vi "Car Wash.vi"(7 "Start":bool, 9 "stop":bool, 10 "Car Position Slider":u8(slide) max=3 scale=0.0..4.0, 11 "Wash Options":T1) -> (0 "error out":errorcluster, 1 "Elapsed Time":dbl format="%0.2f", 2 "Car Wash Indicators":T2, 3 "Wash Entry":bool)   [LabVIEW 2018]
uses:
  Controls/Car Wash Indicators.ctl
  Controls/Wash Options.ctl
  Controls/Car Wash States.ctl
panel:
  out "Array of Control Labels":string[](array[string])
  # "Entry Console"
  # "Car Wash Display"
  # "Car Position Simulation"
  # "Pre-Soak\nH-P Wash\nL-P Wax\nSpot Free Rinse"
  # "Underbody Wash\nBug Remover"
  # "Tire Shine\nAir Dry"
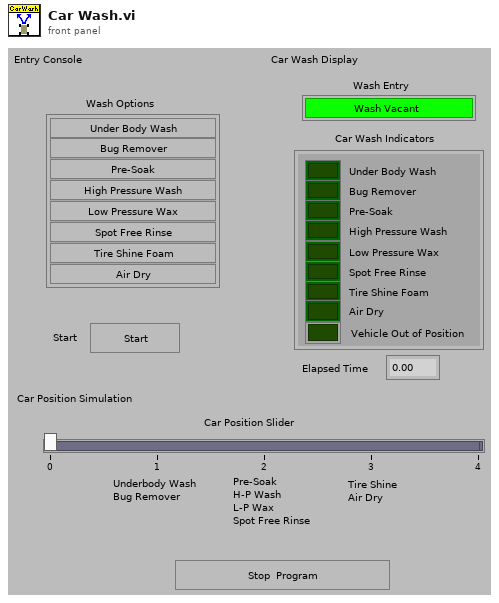
[diagram p1: front panel]
types:
  T1 = typedef "Wash Options.ctl" = cluster{"Underbody Wash":bool, "Bug Remover":bool, "Pre-Soak":bool, "High Pressure Wash":bool, "Low Pressure Wax":bool, "Spot Free Rinse":bool, "Tire Shine Foam":bool, "Air Dry":bool}
  T2 = typedef "Car Wash Indicators.ctl" = cluster{"Under Body Wash":bool, "Bug Remover":bool, "Pre-Soak":bool, "High Pressure Wash":bool, "Low Pressure Wax":bool, "Spot Free Rinse":bool, "Tire Shine Foam":bool, "Air Dry":bool, "Vehicle Out of Position":bool}
  T3 = typedef "Car Wash States.ctl" = enum16{"Initialize", "Customer Select", "Create Wash Process", "Reset Timer", "Under Body Wash", "Bug Remover", "Pre-Soak", "High Pressure Wash", "Low Pressure Wax", "Spot Free Rinse", "Tire Shine Foam", "Air Dry", "Out of Position", "Wash Finished", "Stop"}
  T4 = enum8{"Enabled", "Disabled", "Disabled and Grayed Out"}
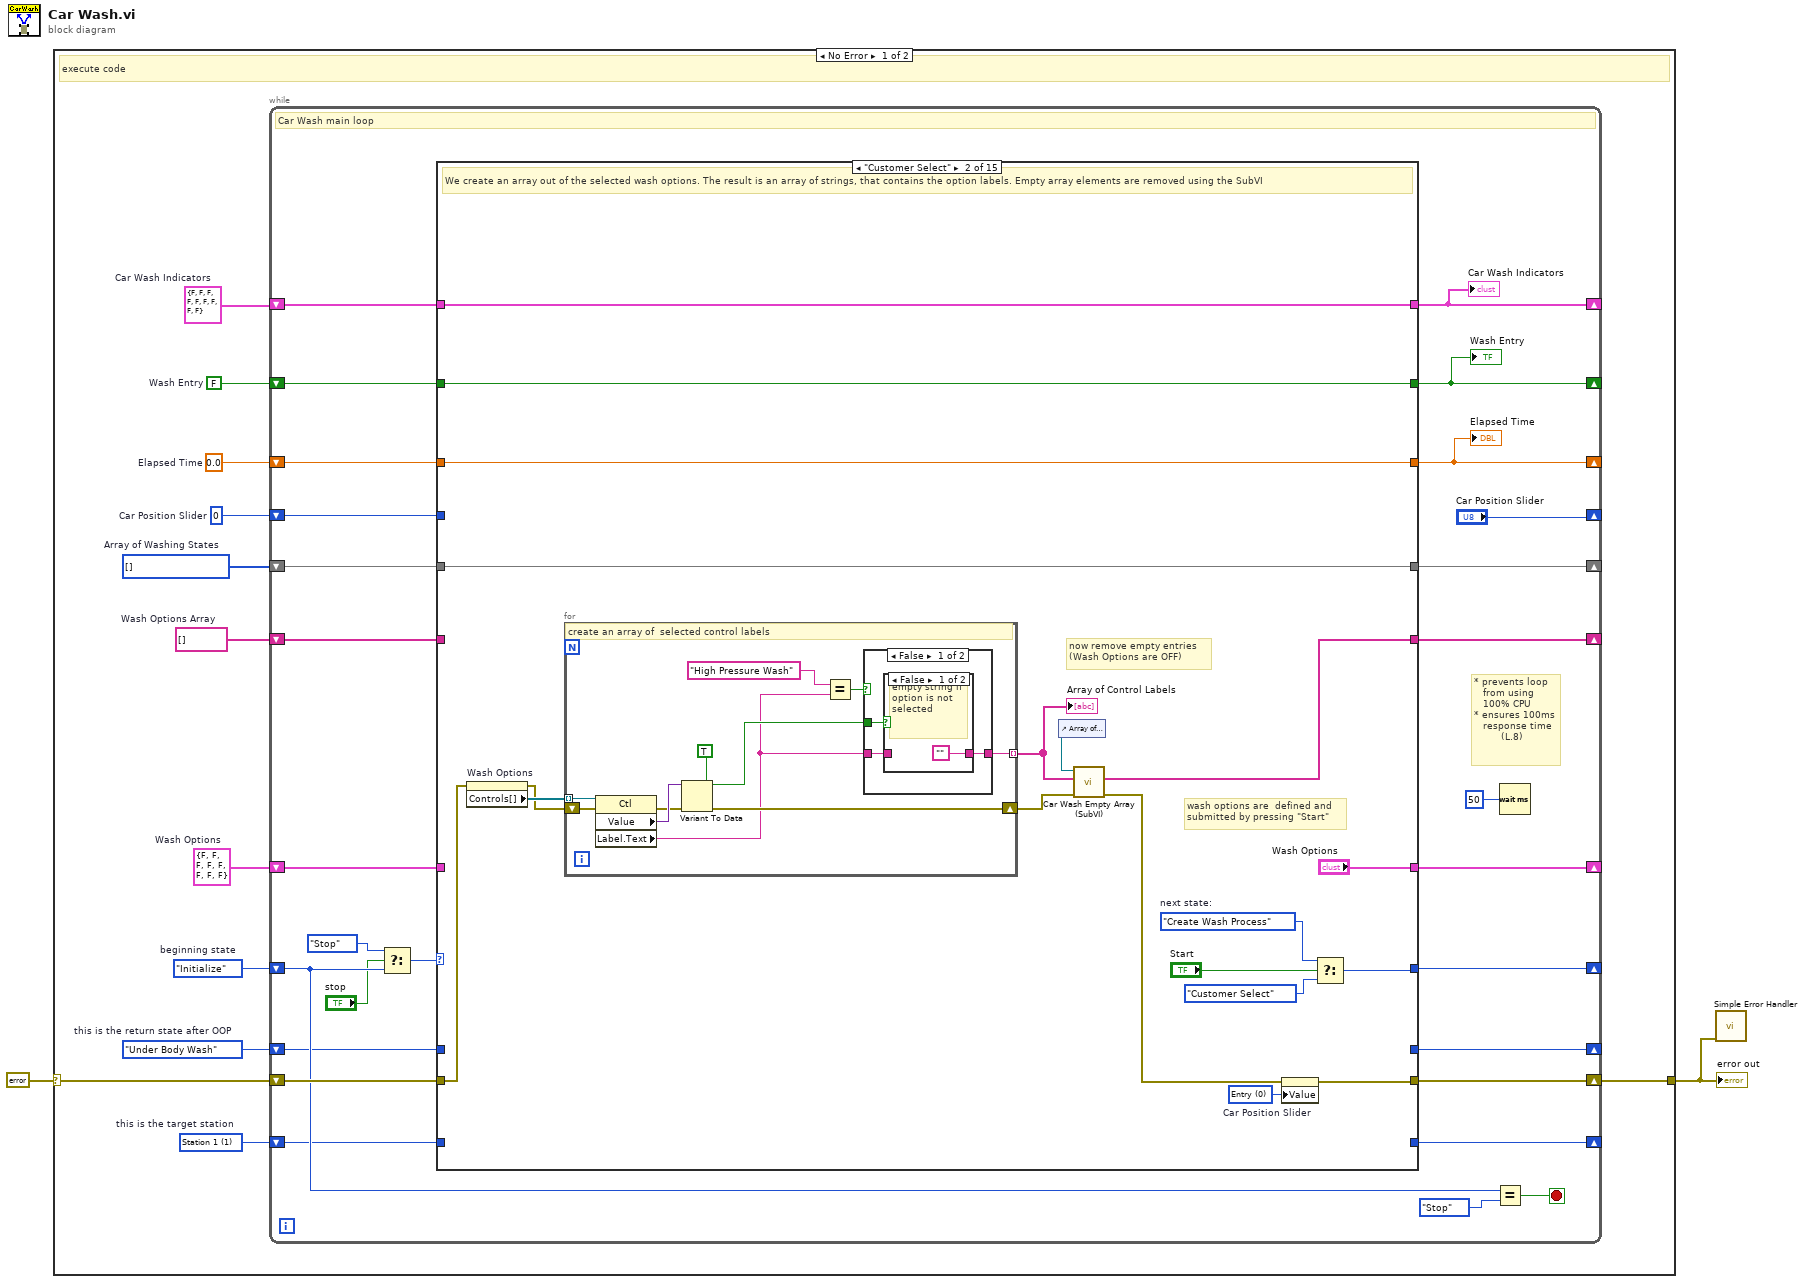
[diagram p0: block diagram]
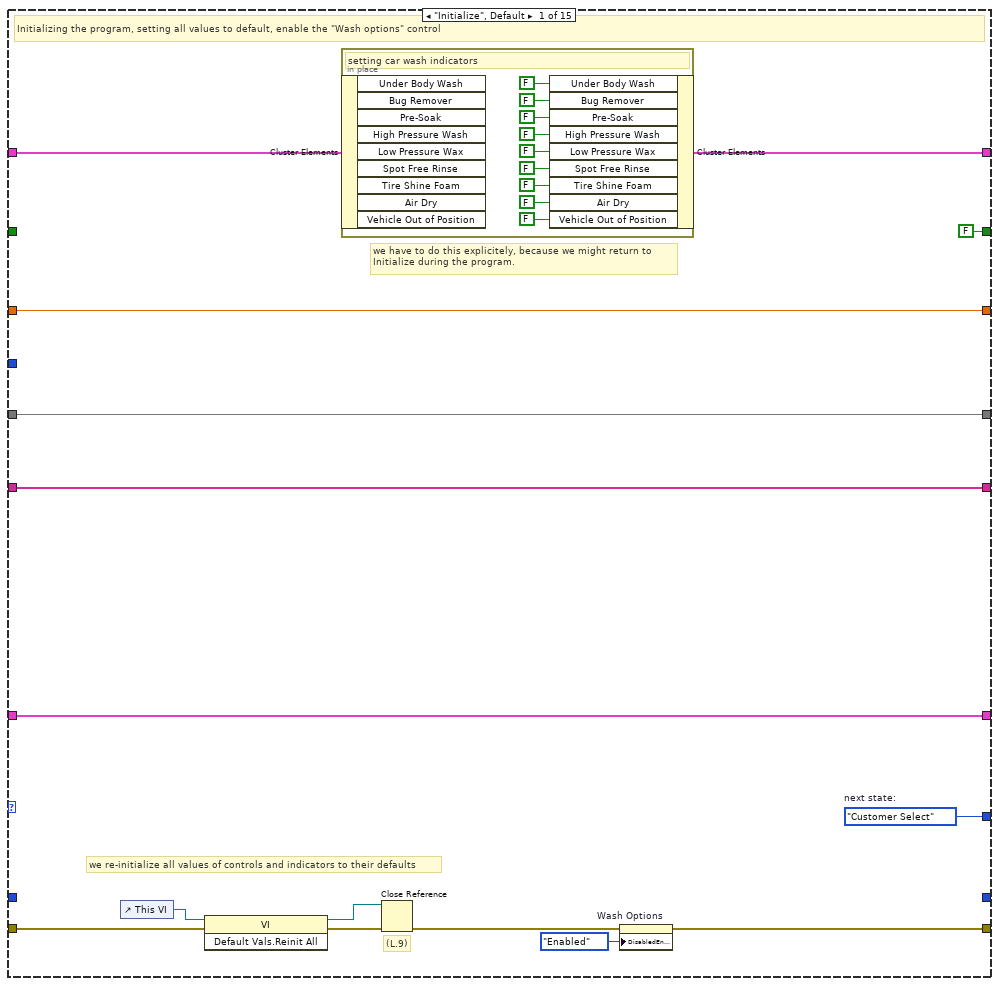
[diagram p2: hidden frame]
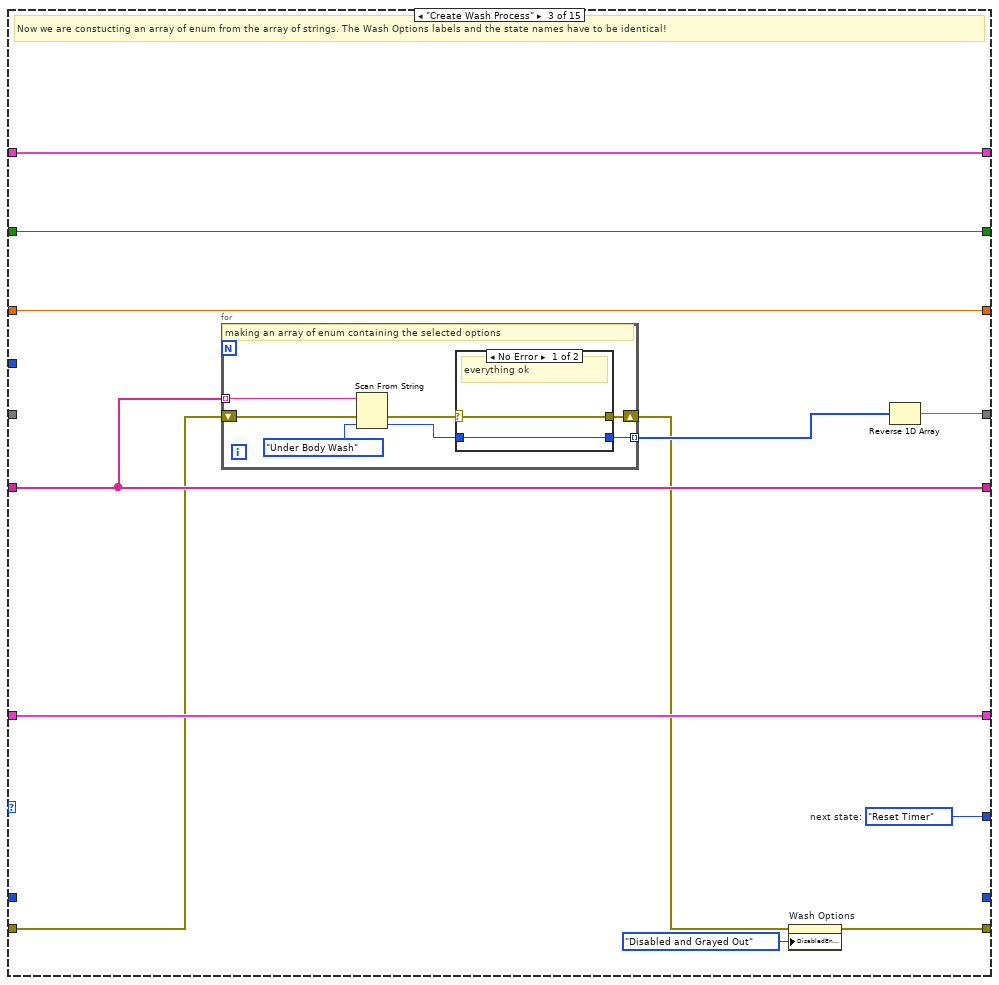
[diagram p5: hidden frame]
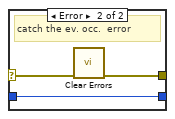
[diagram p6: hidden frame]
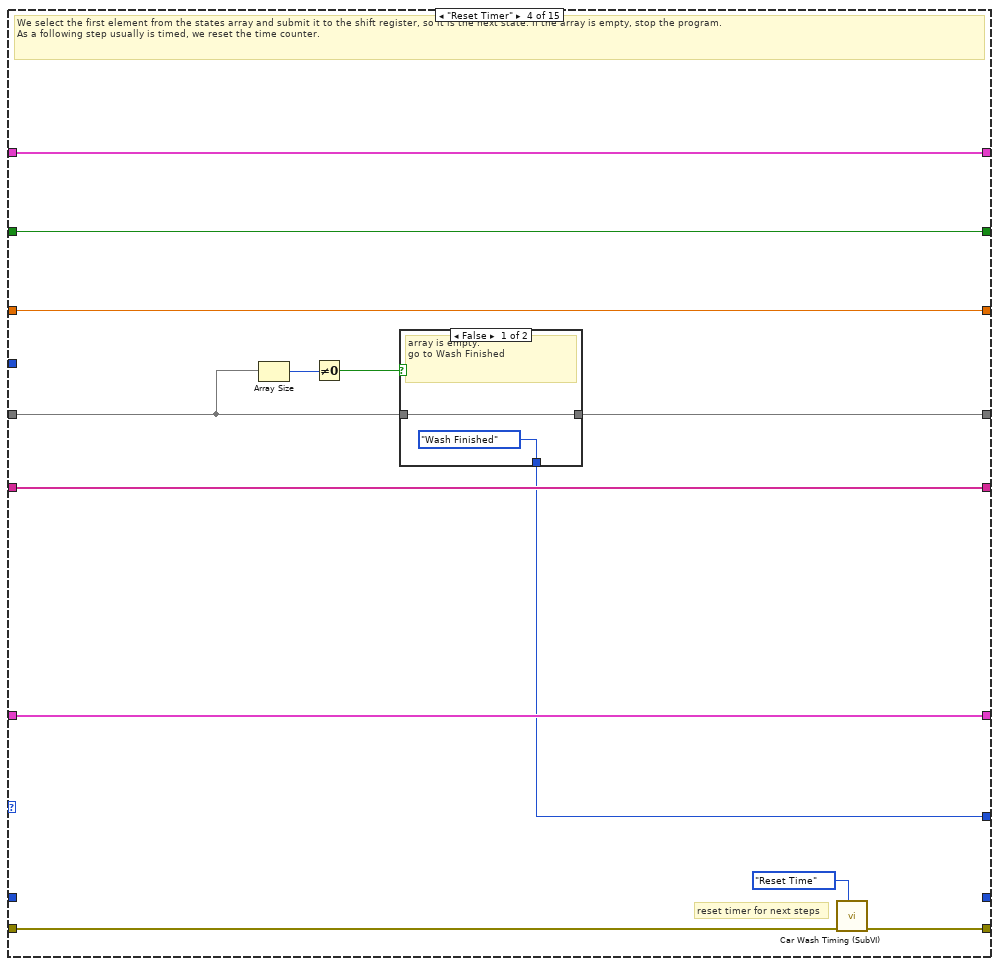
[diagram p7: hidden frame]
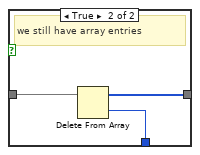
[diagram p8: hidden frame]
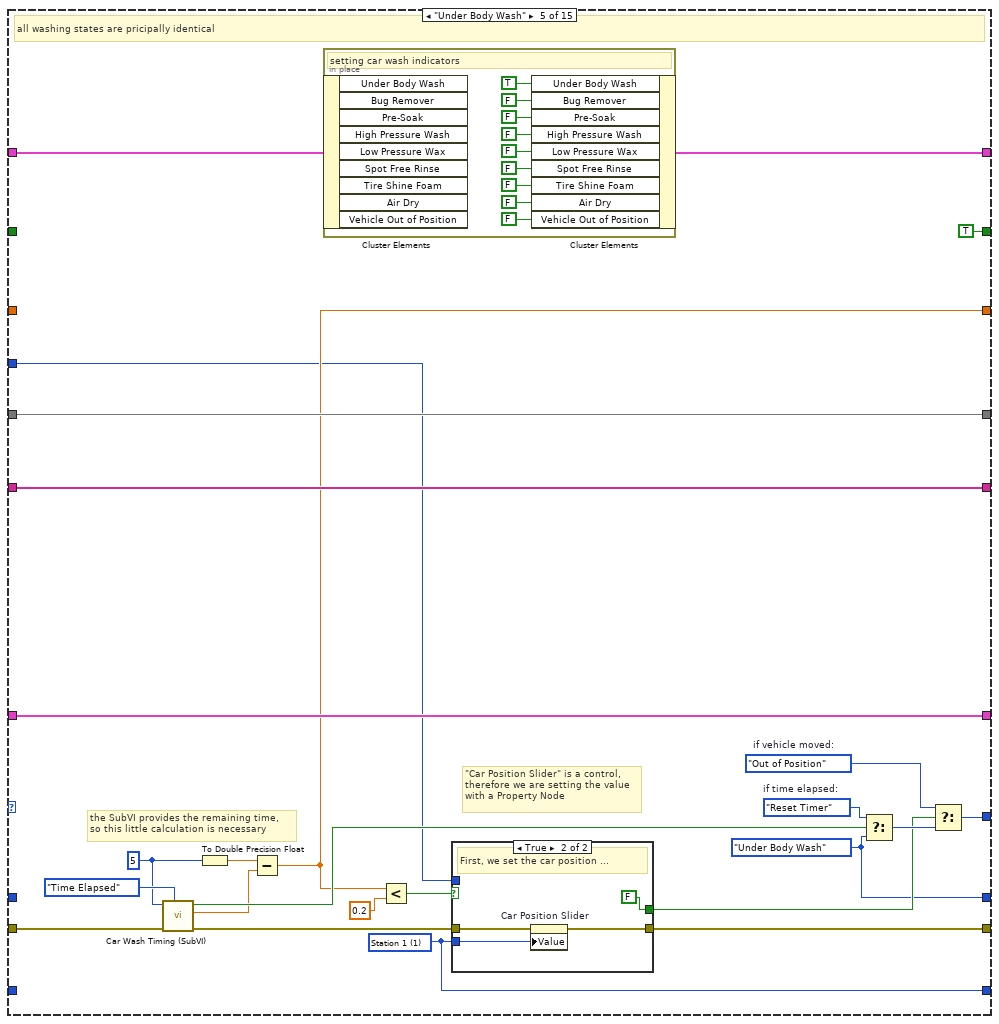
[diagram p9: hidden frame]
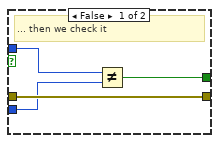
[diagram p10: hidden frame]
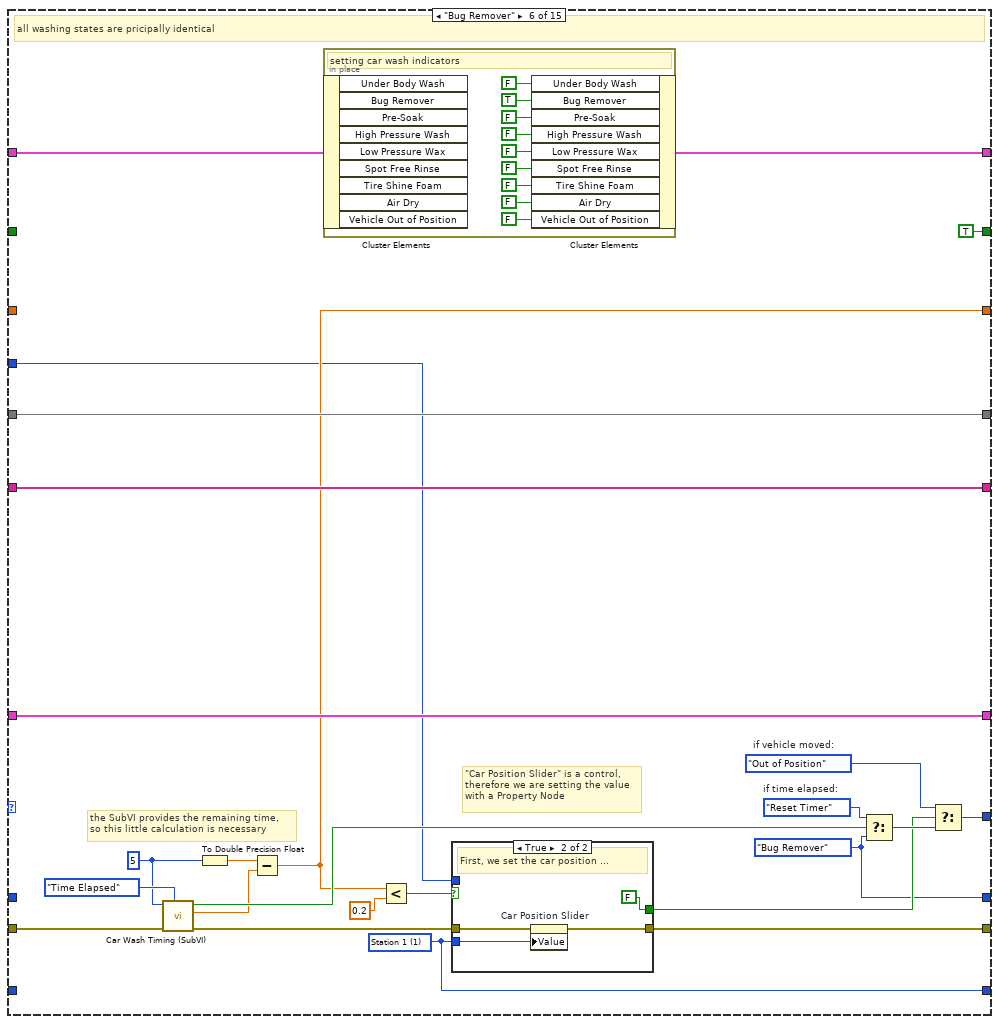
[diagram p11: hidden frame]
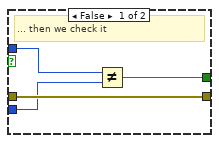
[diagram p12: hidden frame]
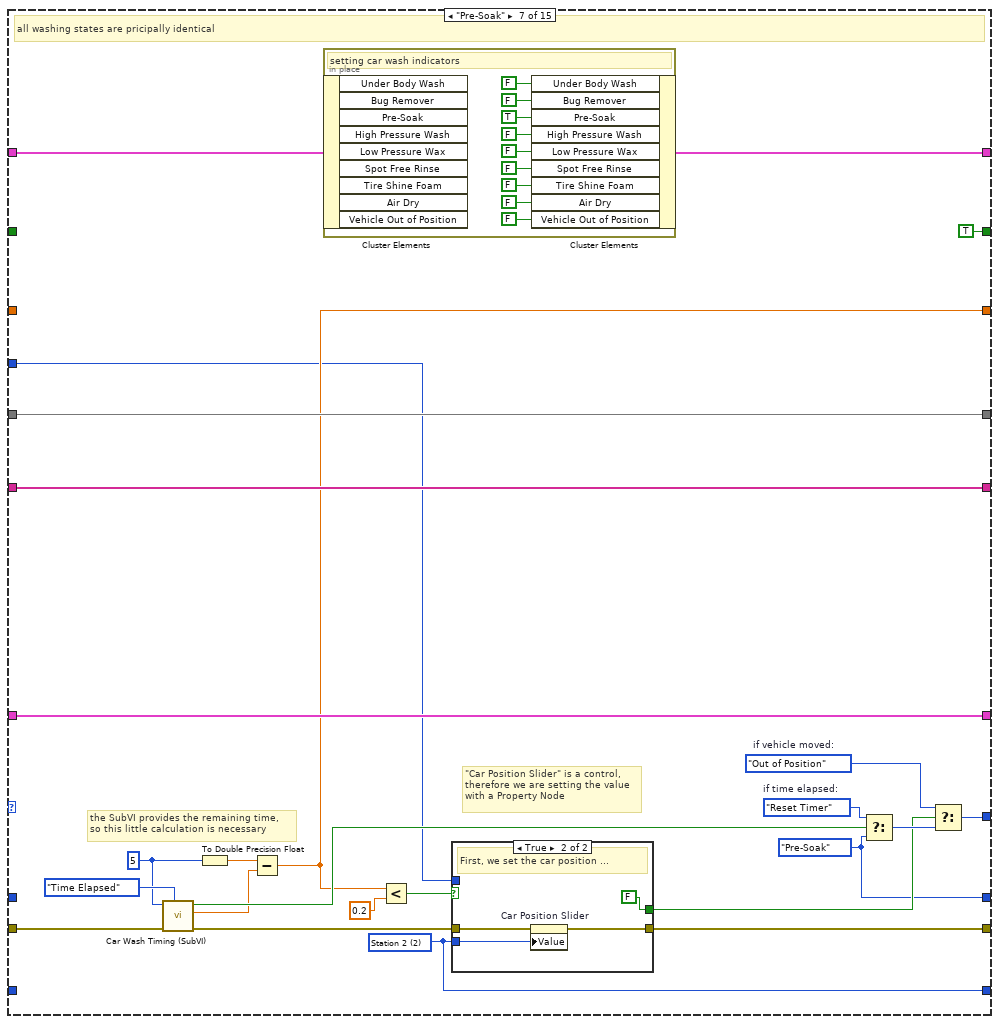
[diagram p13: hidden frame]
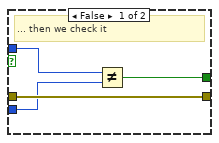
[diagram p14: hidden frame]
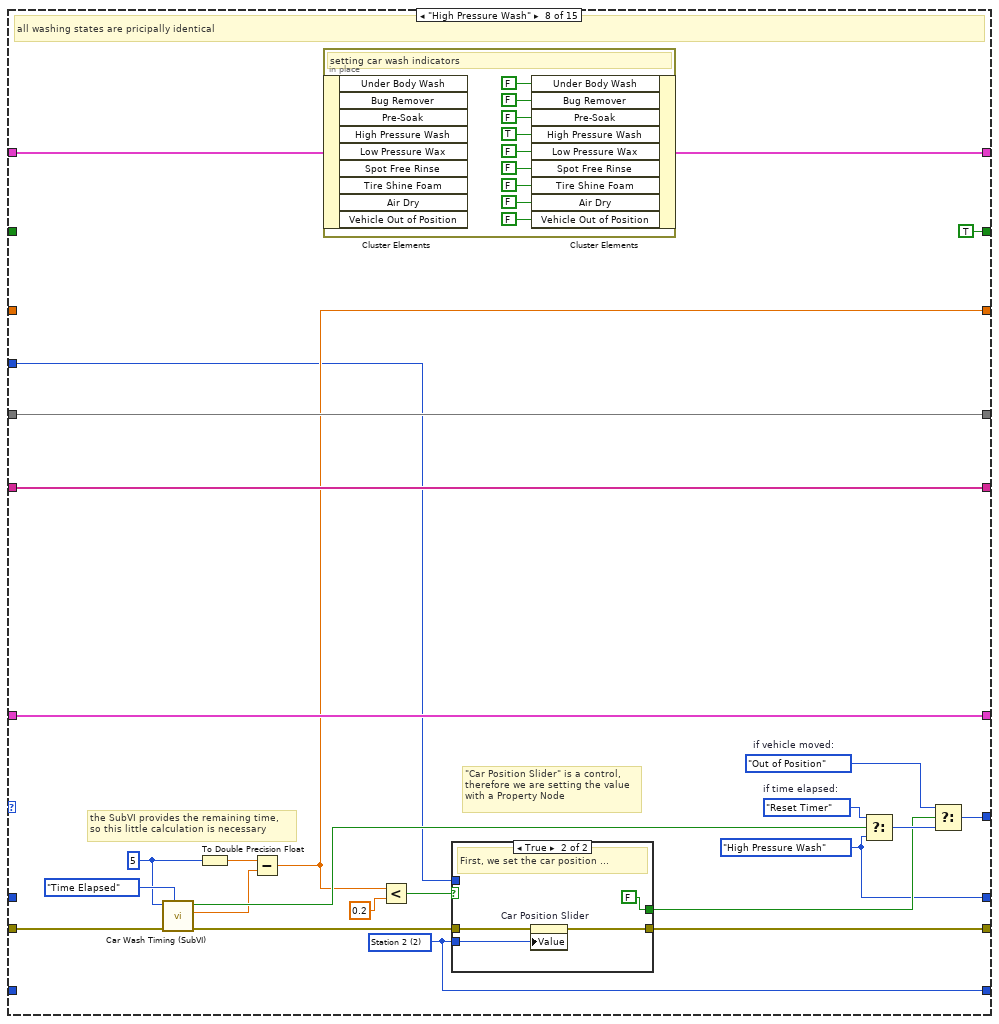
[diagram p15: hidden frame]
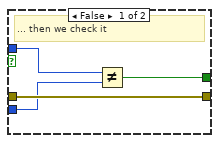
[diagram p16: hidden frame]
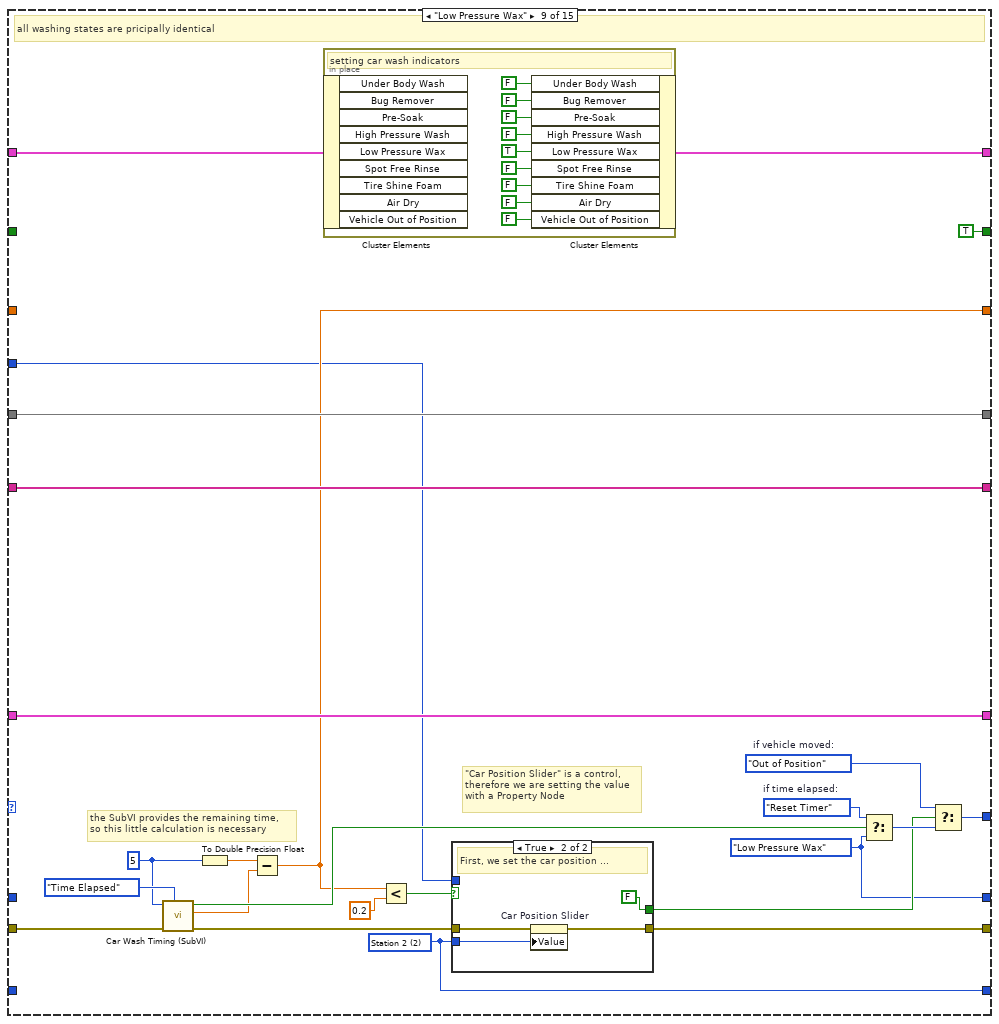
[diagram p17: hidden frame]
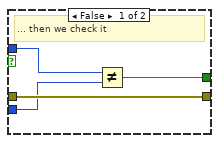
[diagram p18: hidden frame]
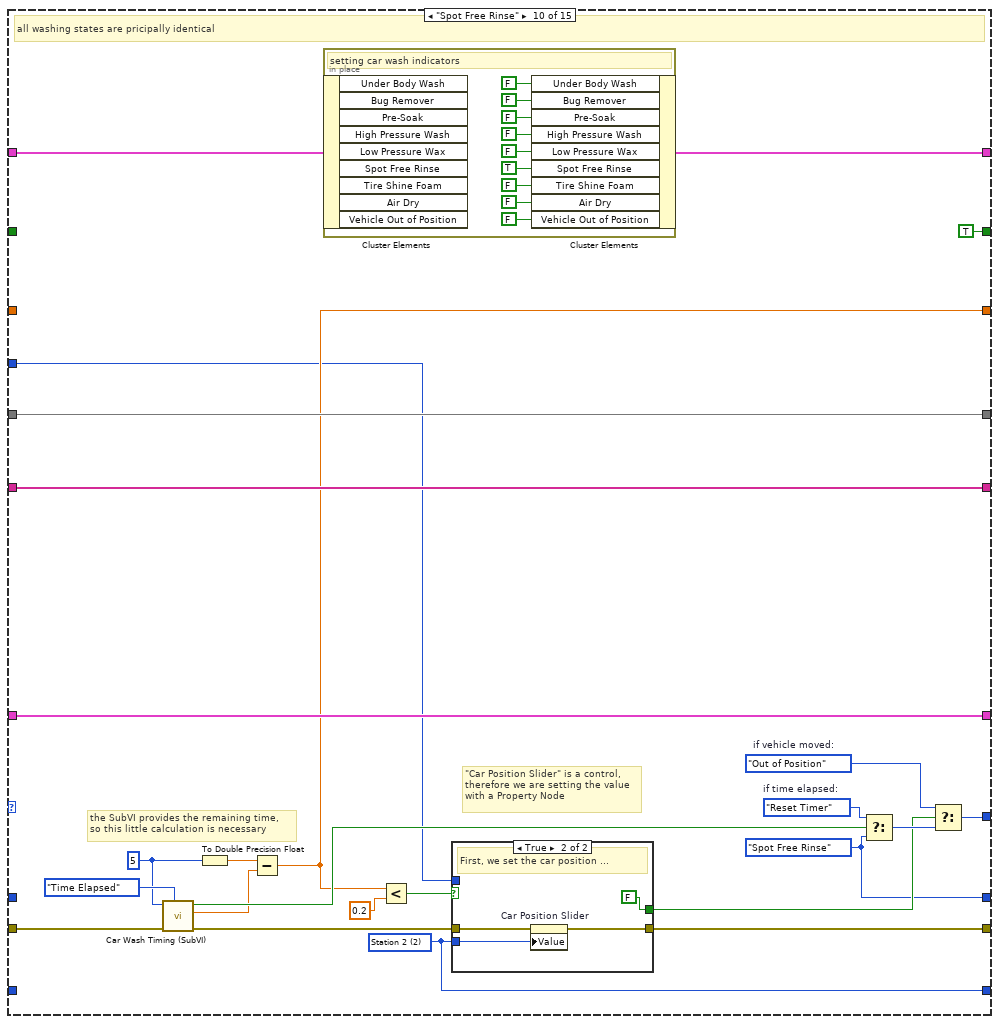
[diagram p19: hidden frame]
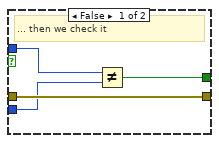
[diagram p20: hidden frame]
diagram:
  n1 = case shown="No Error" errorcluster {"status"=FALSE, "code"=0, "source"=""} ("error in (no error)") {
    selector: errorcluster {"status"=FALSE, "code"=0, "source"=""} ("error in (no error)") -> [w14 w544]
    tunnel: [w13 w544] -> w1
    frame No Error {
      w3 = u8 1 items=["Entry", "Station 1", "Station 2", "Station 3", "Exit"]  # this is the target station
      w4 = Car_Wash_States."Under Body Wash"  # this is the return state after OOP
      w6 = T3[] [] items=["Initialize", "Customer Select", "Create Wash Process", "Reset Timer", "Under Body Wash", "Bug Remover", "Pre-Soak", "High Pressure Wash", "Low Pressure Wax", "Spot Free Rinse", "Tire Shine Foam", "Air Dry", "Out of Position", "Wash Finished", "Stop"]  # Array of Washing States
      w7 = string[] []  # Wash Options Array
      w8 = 0.0  # Elapsed Time
      w9 = FALSE  # Wash Entry
      w10 = T2 {"Under Body Wash"=FALSE, "Bug Remover"=FALSE, "Pre-Soak"=FALSE, "High Pressure Wash"=FALSE, "Low Pressure Wax"=FALSE, "Spot Free Rinse"=FALSE, "Tire Shine Foam"=FALSE, "Air Dry"=FALSE, "Vehicle Out of Position"=FALSE}  # Car Wash Indicators
      w5 = u8 0  # Car Position Slider
      w11 = T1 {"Underbody Wash"=FALSE, "Bug Remover"=FALSE, "Pre-Soak"=FALSE, "High Pressure Wash"=FALSE, "Low Pressure Wax"=FALSE, "Spot Free Rinse"=FALSE, "Tire Shine Foam"=FALSE, "Air Dry"=FALSE}  # Wash Options
      w12 = Car_Wash_States."Initialize"  # beginning state
      # "execute code"
      n2 = while {
        shift-right: [w41] -> w13
        shift-left: w14 -> [w42]
        shift-right: [w25] -> _
        shift-left: w12 -> [w31]
        shift-right: [w37] -> _
        shift-left: w11 -> [w38]
        shift-right: ["Car Position Slider"] -> _
        shift-left: w5 -> [w19]
        shift-right: [w34] -> _
        shift-left: w10 -> [w35]
        shift-right: [w32] -> _
        shift-left: w9 -> [w33]
        shift-right: [w26] -> _
        shift-left: w8 -> [w27]
        shift-right: [w23] -> _
        shift-left: w7 -> [w22]
        shift-right: [w21] -> _
        shift-left: w6 -> [w20]
        shift-right: [w18] -> _
        shift-left: w4 -> [w17]
        shift-right: [w16] -> _
        shift-left: w3 -> [w15]
        stop <- w40 stop-if-true
        # "* prevents loop\n   from using\n   100% CPU\n* ensures 100ms\n   response time\n         (L.8)"
        # "Car Wash main loop"
        n3 = Select(t=Car_Wash_States."Stop", s="stop", f=w31) -> (s? t:f=w30:T3)
        n4 = case shown="\"Customer Select\"" w30 {
          tunnel: w42 -> [w54 w75 w108 w138 w154 w196 w238 w280 w322 w364 w406 w448 w488 w511 w534]
          tunnel: [w43 w69 w104 w139 w149 w191 w233 w275 w317 w359 w401 w443 w488 w505 w529] -> w41
          tunnel: w38 -> [w53 _ w111 w136 w169 w211 w253 w295 w337 w379 w421 w463 w494 w518 w542]
          tunnel: [w53 "Wash Options" w111 w136 w169 w211 w253 w295 w337 w379 w421 w463 w494 w518 w542] -> w37
          tunnel: [w44 w85 w114 w133 w167 w209 w251 w293 w335 w377 w419 w461 w492 w516 w539] -> w34
          tunnel: w35 -> [w45 w85 w114 w133 w168 w210 w252 w294 w336 w378 w420 w462 w493 w517 _]
          tunnel: [FALSE ("Wash Entry") w84 w113 w135 TRUE ("Wash Entry") TRUE ("Wash Entry") TRUE ("Wash Entry") TRUE ("Wash Entry") TRUE ("Wash Entry") TRUE ("Wash Entry") TRUE ("Wash Entry") TRUE ("Wash Entry") TRUE ("Wash Entry") TRUE ("Wash Entry") FALSE ("Wash Entry")] -> w32
          tunnel: w33 -> [_ w84 w113 w135 _ _ _ _ _ _ _ _ _ _ _]
          tunnel: [w52 w83 w112 w134 w152 w194 w236 w278 w320 w362 w404 w446 w487 0.0 ("Elapsed Time") 0.0 ("Elapsed Time")] -> w26
          tunnel: w27 -> [w52 w83 w112 w134 _ _ _ _ _ _ _ _ w487 _ _]
          tunnel: [w51 w82 w110 w130 w157 w199 w241 w283 w325 w367 w409 w451 w486 w512 Car_Wash_States."Stop" ("t")] -> w25
          tunnel: w19 -> [_ _ _ _ w148 w190 w232 w274 w316 w358 w400 w442 w483 _ _]
          tunnel: [w48 w71 w109 w132 w159 w201 w243 w285 w327 w369 w411 w453 w490 w510 string[] [] ("Wash Options Array")] -> w23
          tunnel: w22 -> [w48 _ w109 w132 w159 w201 w243 w285 w327 w369 w411 w453 w490 w510 _]
          tunnel: [w47 w70 w106 w131 w158 w200 w242 w284 w326 w368 w410 w452 w489 w509 w531] -> w21
          tunnel: w20 -> [w47 w70 _ w127 w158 w200 w242 w284 w326 w368 w410 w452 w489 w509 _]
          tunnel: [_ _ _ _ w146 w188 w230 w272 w314 w356 w398 w440 w484 _ _] -> w18
          tunnel: w17 -> [_ _ _ _ _ _ _ _ _ _ _ _ w484 _ _]
          tunnel: [_ _ _ _ w145 w187 w229 w271 w313 w355 w397 w439 w481 _ _] -> w16
          tunnel: w15 -> [_ _ _ _ _ _ _ _ _ _ _ _ w481 _ _]
          frame "Initialize", Default {
            w51 = Car_Wash_States."Customer Select"  # next state:
            # "we have to do this explicitely, because we might return to\nInitialize during the program."
            # "we re-initialize all values of controls and indicators to their defaults"
            # "(L.9)"
            # "Initializing the program, setting all values to default, enable the \"Wash options\" control"
            n5 = control-ref of="This VI"() -> (w57:refnum<vi>)
            n6 = invoke class="VI" method="Default Vals.Reinit All"(reference=w57, error in=w54) -> (reference out=w56:refnum<vi>, error out=w55:errorcluster)  [unwired: 1 in, 1 out]
            n7 = in-place {
              # "setting car wash indicators"
              n8 = in-place-cluster #1(w45) -> ()  [unwired: 9 out]
              n9 = in-place-cluster #1("Under Body Wash"=FALSE, "Bug Remover"=FALSE, "Pre-Soak"=FALSE, "High Pressure Wash"=FALSE, "Low Pressure Wax"=FALSE, "Spot Free Rinse"=FALSE, "Tire Shine Foam"=FALSE, "Air Dry"=FALSE, "Vehicle Out of Position"=FALSE) -> (w44:T2)
            }
            n10 = Close Reference(reference=w56, error in (no error)=w55) -> (error out=w50:errorcluster)
            n11 = property on="Wash Options" class="Clust (strict)"(error in=w50, "DisabledEnum"=T4."Enabled" ("Disabled")) -> (error out=w43:errorcluster)  [unwired: 1 in, 1 out]
          }
          frame "Customer Select" {
            w67 = u8 0 items=["Entry", "Station 1", "Station 2", "Station 3", "Exit"] ("Car Position Slider")
            w81 = Car_Wash_States."Create Wash Process"  # next state:
            # "wash options are  defined and\nsubmitted by pressing \"Start\""
            # "now remove empty entries\n(Wash Options are OFF)"
            # "We create an array out of the selected wash options. The result is an array of strings, that contains the option labels. Empty array elements are removed using the SubVI"
            n12 = property on="Wash Options" class="Clust (strict)"(error in=w75) -> (error out=w76:errorcluster, "Controls[]"=w77:refnum<vi>[])  [unwired: 1 in, 1 out]
            n13 = for {
              tunnel: w77 -> [w96] mode=indexing
              tunnel: [w91] -> w72 mode=indexing
              shift-right: [w89] -> w73
              shift-left: w76 -> [w90]
              # "create an array of  selected control labels"
              n14 = property on="Property Node" class="Ctl"(reference=w96, error in=w90) -> (error out=w92:errorcluster, "Value"=w95:variant, "Label.Text"=w87:string)  [unwired: 1 out]
              n15 = Variant To Data(error in=w92, type=TRUE, Variant=w95) -> (data=w93:bool, error out=w89:errorcluster)
              n16 = Equal?(x="High Pressure Wash" ("y"), y=w87) -> (x = y?=w88:bool)
              n17 = case shown="False" w88 {
                tunnel: w93 -> [w99 _]
                tunnel: [w98 w102] -> w91
                tunnel: w87 -> [w97 w102]
                frame False {
                  n18 = case shown="False" w99 {
                    tunnel: w97 -> [_ w101]
                    tunnel: ["" w101] -> w98
                    frame False {
                      # "empty string if option is not selected"
                    }
                    frame True {
                      # "put control label to array"
                    }
                  }
                }
                frame True {
                  # "This is the default\nwash and always \nadded to the \noptions"
                }
              }
            }
            "Array of Control Labels" <- w72
            n19 = control-ref of="Array of Control Labels"() -> (w74:refnum<vi>)
            n20 = call "Car Wash Empty Array (SubVI).vi"("error in (no error)"=w73, "Array in"=w72, "Array reference in"=w74) -> ("error out"=w68:errorcluster, "Array out"=w71:string[])  [unwired: 6 in, 1 out]
            n21 = property on="Car Position Slider" class="Slide (strict)"(error in=w68, "Value"=w67) -> (error out=w69:errorcluster)  [unwired: 1 in, 1 out]
            n22 = Select(t=w81, s="Start", f=Car_Wash_States."Customer Select") -> (s? t:f=w82:T3)
          }
          frame "Create Wash Process" {
            w110 = Car_Wash_States."Reset Timer"  # next state:
            # "Now we are constucting an array of enum from the array of strings. The Wash Options labels and the state names have to be identical!"
            n23 = for {
              tunnel: w109 -> [w121] mode=indexing
              tunnel: [w117] -> w107 mode=indexing
              shift-right: [w115] -> w105
              shift-left: w108 -> [w119]
              # "making an array of enum containing the selected options"
              n24 = Scan From String "Scan From String"(input string=w121, error in=w119, default 1=Car_Wash_States."Under Body Wash" ("beginning state")) -> (error out=w118:errorcluster, output 1=w116:T3)  [unwired: 2 in, 2 out]
              n25 = case shown="No Error" w118 {
                selector: w118 -> [w122 w125]
                tunnel: [w123 w126] -> w117
                tunnel: w116 -> [w123 w126]
                tunnel: [w122 w124] -> w115
                frame No Error {
                  # "everything ok"
                }
                frame Error {
                  # "catch the ev. occ.  error"
                  n26 = call <vilib>:"Clear Errors.vi"("error in (no error)"=w125) -> ("error out"=w124:errorcluster)  [unwired: 5 in, 1 out]
                }
              }
            }
            n27 = property on="Wash Options" class="Clust (strict)"(error in=w105, "DisabledEnum"=T4."Disabled and Grayed Out" ("Disabled")) -> (error out=w104:errorcluster)  [unwired: 1 in, 1 out]
            n28 = Reverse 1D Array(array=w107) -> (reversed array=w106:T3[])
          }
          frame "Reset Timer" {
            # "reset timer for next steps"
            # "We select the first element from the states array and submit it to the shift register, so it is the next state. If the array is empty, stop the program. \nAs a following step usually is timed, we reset the time counter."
            n29 = Array Size(array=w127) -> (size(s)=w129:i32)
            n30 = Not Equal To 0?(x=w129) -> (x != 0?=w128:bool)
            n31 = case shown="False" w128 {
              tunnel: [w141 w144] -> w131
              tunnel: [Car_Wash_States."Wash Finished" ("beginning state") w143] -> w130
              tunnel: w127 -> [w141 w142]
              frame False {
                # "array is empty: \ngo to Wash Finished"
              }
              frame True {
                # "we still have array entries"
                n32 = Delete From Array "Delete From Array"(array=w142) -> (deleted portion=w143:T3, array with subset deleted=w144:T3[])  [unwired: 2 in]
              }
            }
            n33 = call "Car Wash Timing (SubVI).vi"("Function"=enum16{"Reset Time", "Time Elapsed"}."Reset Time", "error in (no error)"=w138) -> ("error out"=w139:errorcluster)  [unwired: 7 in, 2 out]
          }
          frame "Under Body Wash" {
            w145 = u8 1 items=["Entry", "Station 1", "Station 2", "Station 3", "Exit"] ("Car Position Slider")
            w155 = Car_Wash_States."Out of Position"  # if vehicle moved:
            w146 = Car_Wash_States."Under Body Wash" ("t")
            w164 = Car_Wash_States."Reset Timer"  # if time elapsed:
            w160 = 5 ("Time to Wait (s)")
            # "\"Car Position Slider\" is a control,\ntherefore we are setting the value\nwith a Property Node"
            # "the SubVI provides the remaining time,\nso this little calculation is necessary"
            # "all washing states are pricipally identical"
            n34 = call "Car Wash Timing (SubVI).vi"("Function"=enum16{"Reset Time", "Time Elapsed"}."Time Elapsed", "error in (no error)"=w154, "Time to Wait (s)"=w160) -> ("error out"=w150:errorcluster, "Remaining Time"=w162:dbl, "Time elapsed ?"=w163:bool)  [unwired: 6 in]
            n35 = To Double Precision Float(number=w160) -> (double precision float=w161:dbl)
            n36 = Subtract(x=w161, y=w162) -> (x-y=w152:dbl)
            n37 = in-place {
              # "setting car wash indicators"
              n38 = in-place-cluster #2(w168) -> ()  [unwired: 9 out]
              n39 = in-place-cluster #2("Under Body Wash"=TRUE, "Bug Remover"=FALSE, "Pre-Soak"=FALSE, "High Pressure Wash"=FALSE, "Low Pressure Wax"=FALSE, "Spot Free Rinse"=FALSE, "Tire Shine Foam"=FALSE, "Air Dry"=FALSE, "Vehicle Out of Position"=FALSE) -> (w167:T2)
            }
            n40 = Less?(x=w152, y=0.2) -> (x < y?=w151:bool)
            n41 = case shown="True" w151 {
              tunnel: w150 -> [w173 w177]
              tunnel: [w173 w176] -> w149
              tunnel: w145 -> [w170 w175]
              tunnel: w148 -> [w172 _]
              tunnel: [w171 FALSE] -> w147
              frame False {
                # "... then we check it"
                n42 = Not Equal?(x=w172, y=w170) -> (x != y?=w171:bool)
              }
              frame True {
                # "First, we set the car position ..."
                n43 = property on="Car Position Slider" class="Slide (strict)"(error in=w177, "Value"=w175) -> (error out=w176:errorcluster)  [unwired: 1 in, 1 out]
              }
            }
            n44 = Select(t=w164, s=w163, f=w146) -> (s? t:f=w156:T3)
            n45 = Select(t=w155, s=w147, f=w156) -> (s? t:f=w157:T3)
          }
          frame "Bug Remover" {
            w187 = u8 1 items=["Entry", "Station 1", "Station 2", "Station 3", "Exit"] ("Car Position Slider")
            w197 = Car_Wash_States."Out of Position"  # if vehicle moved:
            w188 = Car_Wash_States."Bug Remover" ("t")
            w206 = Car_Wash_States."Reset Timer"  # if time elapsed:
            w202 = 5 ("Time to Wait (s)")
            # "\"Car Position Slider\" is a control,\ntherefore we are setting the value\nwith a Property Node"
            # "the SubVI provides the remaining time,\nso this little calculation is necessary"
            # "all washing states are pricipally identical"
            n46 = call "Car Wash Timing (SubVI).vi"("Function"=enum16{"Reset Time", "Time Elapsed"}."Time Elapsed", "error in (no error)"=w196, "Time to Wait (s)"=w202) -> ("error out"=w192:errorcluster, "Remaining Time"=w204:dbl, "Time elapsed ?"=w205:bool)  [unwired: 6 in]
            n47 = To Double Precision Float(number=w202) -> (double precision float=w203:dbl)
            n48 = Subtract(x=w203, y=w204) -> (x-y=w194:dbl)
            n49 = in-place {
              # "setting car wash indicators"
              n50 = in-place-cluster #3(w210) -> ()  [unwired: 9 out]
              n51 = in-place-cluster #3("Under Body Wash"=FALSE, "Bug Remover"=TRUE, "Pre-Soak"=FALSE, "High Pressure Wash"=FALSE, "Low Pressure Wax"=FALSE, "Spot Free Rinse"=FALSE, "Tire Shine Foam"=FALSE, "Air Dry"=FALSE, "Vehicle Out of Position"=FALSE) -> (w209:T2)
            }
            n52 = Less?(x=w194, y=0.2) -> (x < y?=w193:bool)
            n53 = case shown="True" w193 {
              tunnel: w192 -> [w215 w219]
              tunnel: [w215 w218] -> w191
              tunnel: w187 -> [w212 w217]
              tunnel: w190 -> [w214 _]
              tunnel: [w213 FALSE] -> w189
              frame False {
                # "... then we check it"
                n54 = Not Equal?(x=w214, y=w212) -> (x != y?=w213:bool)
              }
              frame True {
                # "First, we set the car position ..."
                n55 = property on="Car Position Slider" class="Slide (strict)"(error in=w219, "Value"=w217) -> (error out=w218:errorcluster)  [unwired: 1 in, 1 out]
              }
            }
            n56 = Select(t=w206, s=w205, f=w188) -> (s? t:f=w198:T3)
            n57 = Select(t=w197, s=w189, f=w198) -> (s? t:f=w199:T3)
          }
          frame "Pre-Soak" {
            w229 = u8 2 items=["Entry", "Station 1", "Station 2", "Station 3", "Exit"] ("Car Position Slider")
            w239 = Car_Wash_States."Out of Position"  # if vehicle moved:
            w230 = Car_Wash_States."Pre-Soak" ("t")
            w248 = Car_Wash_States."Reset Timer"  # if time elapsed:
            w244 = 5 ("Time to Wait (s)")
            # "\"Car Position Slider\" is a control,\ntherefore we are setting the value\nwith a Property Node"
            # "the SubVI provides the remaining time,\nso this little calculation is necessary"
            # "all washing states are pricipally identical"
            n58 = call "Car Wash Timing (SubVI).vi"("Function"=enum16{"Reset Time", "Time Elapsed"}."Time Elapsed", "error in (no error)"=w238, "Time to Wait (s)"=w244) -> ("error out"=w234:errorcluster, "Remaining Time"=w246:dbl, "Time elapsed ?"=w247:bool)  [unwired: 6 in]
            n59 = To Double Precision Float(number=w244) -> (double precision float=w245:dbl)
            n60 = Subtract(x=w245, y=w246) -> (x-y=w236:dbl)
            n61 = in-place {
              # "setting car wash indicators"
              n62 = in-place-cluster #4(w252) -> ()  [unwired: 9 out]
              n63 = in-place-cluster #4("Under Body Wash"=FALSE, "Bug Remover"=FALSE, "Pre-Soak"=TRUE, "High Pressure Wash"=FALSE, "Low Pressure Wax"=FALSE, "Spot Free Rinse"=FALSE, "Tire Shine Foam"=FALSE, "Air Dry"=FALSE, "Vehicle Out of Position"=FALSE) -> (w251:T2)
            }
            n64 = Less?(x=w236, y=0.2) -> (x < y?=w235:bool)
            n65 = case shown="True" w235 {
              tunnel: w234 -> [w257 w261]
              tunnel: [w257 w260] -> w233
              tunnel: w229 -> [w254 w259]
              tunnel: w232 -> [w256 _]
              tunnel: [w255 FALSE] -> w231
              frame False {
                # "... then we check it"
                n66 = Not Equal?(x=w256, y=w254) -> (x != y?=w255:bool)
              }
              frame True {
                # "First, we set the car position ..."
                n67 = property on="Car Position Slider" class="Slide (strict)"(error in=w261, "Value"=w259) -> (error out=w260:errorcluster)  [unwired: 1 in, 1 out]
              }
            }
            n68 = Select(t=w248, s=w247, f=w230) -> (s? t:f=w240:T3)
            n69 = Select(t=w239, s=w231, f=w240) -> (s? t:f=w241:T3)
          }
          frame "High Pressure Wash" {
            w271 = u8 2 items=["Entry", "Station 1", "Station 2", "Station 3", "Exit"] ("Car Position Slider")
            w281 = Car_Wash_States."Out of Position"  # if vehicle moved:
            w272 = Car_Wash_States."High Pressure Wash" ("t")
            w290 = Car_Wash_States."Reset Timer"  # if time elapsed:
            w286 = 5 ("Time to Wait (s)")
            # "\"Car Position Slider\" is a control,\ntherefore we are setting the value\nwith a Property Node"
            # "the SubVI provides the remaining time,\nso this little calculation is necessary"
            # "all washing states are pricipally identical"
            n70 = call "Car Wash Timing (SubVI).vi"("Function"=enum16{"Reset Time", "Time Elapsed"}."Time Elapsed", "error in (no error)"=w280, "Time to Wait (s)"=w286) -> ("error out"=w276:errorcluster, "Remaining Time"=w288:dbl, "Time elapsed ?"=w289:bool)  [unwired: 6 in]
            n71 = To Double Precision Float(number=w286) -> (double precision float=w287:dbl)
            n72 = Subtract(x=w287, y=w288) -> (x-y=w278:dbl)
            n73 = in-place {
              # "setting car wash indicators"
              n74 = in-place-cluster #5(w294) -> ()  [unwired: 9 out]
              n75 = in-place-cluster #5("Under Body Wash"=FALSE, "Bug Remover"=FALSE, "Pre-Soak"=FALSE, "High Pressure Wash"=TRUE, "Low Pressure Wax"=FALSE, "Spot Free Rinse"=FALSE, "Tire Shine Foam"=FALSE, "Air Dry"=FALSE, "Vehicle Out of Position"=FALSE) -> (w293:T2)
            }
            n76 = Less?(x=w278, y=0.2) -> (x < y?=w277:bool)
            n77 = case shown="True" w277 {
              tunnel: w276 -> [w299 w303]
              tunnel: [w299 w302] -> w275
              tunnel: w271 -> [w296 w301]
              tunnel: w274 -> [w298 _]
              tunnel: [w297 FALSE] -> w273
              frame False {
                # "... then we check it"
                n78 = Not Equal?(x=w298, y=w296) -> (x != y?=w297:bool)
              }
              frame True {
                # "First, we set the car position ..."
                n79 = property on="Car Position Slider" class="Slide (strict)"(error in=w303, "Value"=w301) -> (error out=w302:errorcluster)  [unwired: 1 in, 1 out]
              }
            }
            n80 = Select(t=w290, s=w289, f=w272) -> (s? t:f=w282:T3)
            n81 = Select(t=w281, s=w273, f=w282) -> (s? t:f=w283:T3)
          }
          frame "Low Pressure Wax" {
            w313 = u8 2 items=["Entry", "Station 1", "Station 2", "Station 3", "Exit"] ("Car Position Slider")
            w323 = Car_Wash_States."Out of Position"  # if vehicle moved:
            w314 = Car_Wash_States."Low Pressure Wax" ("t")
            w332 = Car_Wash_States."Reset Timer"  # if time elapsed:
            w328 = 5 ("Time to Wait (s)")
            # "\"Car Position Slider\" is a control,\ntherefore we are setting the value\nwith a Property Node"
            # "the SubVI provides the remaining time,\nso this little calculation is necessary"
            # "all washing states are pricipally identical"
            n82 = call "Car Wash Timing (SubVI).vi"("Function"=enum16{"Reset Time", "Time Elapsed"}."Time Elapsed", "error in (no error)"=w322, "Time to Wait (s)"=w328) -> ("error out"=w318:errorcluster, "Remaining Time"=w330:dbl, "Time elapsed ?"=w331:bool)  [unwired: 6 in]
            n83 = To Double Precision Float(number=w328) -> (double precision float=w329:dbl)
            n84 = Subtract(x=w329, y=w330) -> (x-y=w320:dbl)
            n85 = in-place {
              # "setting car wash indicators"
              n86 = in-place-cluster #6(w336) -> ()  [unwired: 9 out]
              n87 = in-place-cluster #6("Under Body Wash"=FALSE, "Bug Remover"=FALSE, "Pre-Soak"=FALSE, "High Pressure Wash"=FALSE, "Low Pressure Wax"=TRUE, "Spot Free Rinse"=FALSE, "Tire Shine Foam"=FALSE, "Air Dry"=FALSE, "Vehicle Out of Position"=FALSE) -> (w335:T2)
            }
            n88 = Less?(x=w320, y=0.2) -> (x < y?=w319:bool)
            n89 = case shown="True" w319 {
              tunnel: w318 -> [w341 w345]
              tunnel: [w341 w344] -> w317
              tunnel: w313 -> [w338 w343]
              tunnel: w316 -> [w340 _]
              tunnel: [w339 FALSE] -> w315
              frame False {
                # "... then we check it"
                n90 = Not Equal?(x=w340, y=w338) -> (x != y?=w339:bool)
              }
              frame True {
                # "First, we set the car position ..."
                n91 = property on="Car Position Slider" class="Slide (strict)"(error in=w345, "Value"=w343) -> (error out=w344:errorcluster)  [unwired: 1 in, 1 out]
              }
            }
            n92 = Select(t=w332, s=w331, f=w314) -> (s? t:f=w324:T3)
            n93 = Select(t=w323, s=w315, f=w324) -> (s? t:f=w325:T3)
          }
          frame "Spot Free Rinse" {
            w355 = u8 2 items=["Entry", "Station 1", "Station 2", "Station 3", "Exit"] ("Car Position Slider")
            w365 = Car_Wash_States."Out of Position"  # if vehicle moved:
            w356 = Car_Wash_States."Spot Free Rinse" ("t")
            w374 = Car_Wash_States."Reset Timer"  # if time elapsed:
            w370 = 5 ("Time to Wait (s)")
            # "\"Car Position Slider\" is a control,\ntherefore we are setting the value\nwith a Property Node"
            # "the SubVI provides the remaining time,\nso this little calculation is necessary"
            # "all washing states are pricipally identical"
            n94 = call "Car Wash Timing (SubVI).vi"("Function"=enum16{"Reset Time", "Time Elapsed"}."Time Elapsed", "error in (no error)"=w364, "Time to Wait (s)"=w370) -> ("error out"=w360:errorcluster, "Remaining Time"=w372:dbl, "Time elapsed ?"=w373:bool)  [unwired: 6 in]
            n95 = To Double Precision Float(number=w370) -> (double precision float=w371:dbl)
            n96 = Subtract(x=w371, y=w372) -> (x-y=w362:dbl)
            n97 = in-place {
              # "setting car wash indicators"
              n98 = in-place-cluster #7(w378) -> ()  [unwired: 9 out]
              n99 = in-place-cluster #7("Under Body Wash"=FALSE, "Bug Remover"=FALSE, "Pre-Soak"=FALSE, "High Pressure Wash"=FALSE, "Low Pressure Wax"=FALSE, "Spot Free Rinse"=TRUE, "Tire Shine Foam"=FALSE, "Air Dry"=FALSE, "Vehicle Out of Position"=FALSE) -> (w377:T2)
            }
            n100 = Less?(x=w362, y=0.2) -> (x < y?=w361:bool)
            n101 = case shown="True" w361 {
              tunnel: w360 -> [w383 w387]
              tunnel: [w383 w386] -> w359
              tunnel: w355 -> [w380 w385]
              tunnel: w358 -> [w382 _]
              tunnel: [w381 FALSE] -> w357
              frame False {
                # "... then we check it"
                n102 = Not Equal?(x=w382, y=w380) -> (x != y?=w381:bool)
              }
              frame True {
                # "First, we set the car position ..."
                n103 = property on="Car Position Slider" class="Slide (strict)"(error in=w387, "Value"=w385) -> (error out=w386:errorcluster)  [unwired: 1 in, 1 out]
              }
            }
            n104 = Select(t=w374, s=w373, f=w356) -> (s? t:f=w366:T3)
            n105 = Select(t=w365, s=w357, f=w366) -> (s? t:f=w367:T3)
          }
          frame "Tire Shine Foam" {
            w397 = u8 3 items=["Entry", "Station 1", "Station 2", "Station 3", "Exit"] ("Car Position Slider")
            w407 = Car_Wash_States."Out of Position"  # if vehicle moved:
            w398 = Car_Wash_States."Tire Shine Foam" ("t")
            w416 = Car_Wash_States."Reset Timer"  # if time elapsed:
            w412 = 5 ("Time to Wait (s)")
            # "\"Car Position Slider\" is a control,\ntherefore we are setting the value\nwith a Property Node"
            # "the SubVI provides the remaining time,\nso this little calculation is necessary"
            # "all washing states are pricipally identical"
            n106 = call "Car Wash Timing (SubVI).vi"("Function"=enum16{"Reset Time", "Time Elapsed"}."Time Elapsed", "error in (no error)"=w406, "Time to Wait (s)"=w412) -> ("error out"=w402:errorcluster, "Remaining Time"=w414:dbl, "Time elapsed ?"=w415:bool)  [unwired: 6 in]
            n107 = To Double Precision Float(number=w412) -> (double precision float=w413:dbl)
            n108 = Subtract(x=w413, y=w414) -> (x-y=w404:dbl)
            n109 = in-place {
              # "setting car wash indicators"
              n110 = in-place-cluster #8(w420) -> ()  [unwired: 9 out]
              n111 = in-place-cluster #8("Under Body Wash"=FALSE, "Bug Remover"=FALSE, "Pre-Soak"=FALSE, "High Pressure Wash"=FALSE, "Low Pressure Wax"=FALSE, "Spot Free Rinse"=FALSE, "Tire Shine Foam"=TRUE, "Air Dry"=FALSE, "Vehicle Out of Position"=FALSE) -> (w419:T2)
            }
            n112 = Less?(x=w404, y=0.2) -> (x < y?=w403:bool)
            n113 = case shown="True" w403 {
              tunnel: w402 -> [w425 w429]
              tunnel: [w425 w428] -> w401
              tunnel: w397 -> [w422 w427]
              tunnel: w400 -> [w424 _]
              tunnel: [w423 FALSE] -> w399
              frame False {
                # "... then we check it"
                n114 = Not Equal?(x=w424, y=w422) -> (x != y?=w423:bool)
              }
              frame True {
                # "First, we set the car position ..."
                n115 = property on="Car Position Slider" class="Slide (strict)"(error in=w429, "Value"=w427) -> (error out=w428:errorcluster)  [unwired: 1 in, 1 out]
              }
            }
            n116 = Select(t=w416, s=w415, f=w398) -> (s? t:f=w408:T3)
            n117 = Select(t=w407, s=w399, f=w408) -> (s? t:f=w409:T3)
          }
          frame "Air Dry" {
            w439 = u8 3 items=["Entry", "Station 1", "Station 2", "Station 3", "Exit"] ("Car Position Slider")
            w449 = Car_Wash_States."Out of Position"  # if vehicle moved:
            w440 = Car_Wash_States."Air Dry" ("t")
            w458 = Car_Wash_States."Reset Timer"  # if time elapsed:
            w454 = 5 ("Time to Wait (s)")
            # "\"Car Position Slider\" is a control,\ntherefore we are setting the value\nwith a Property Node"
            # "the SubVI provides the remaining time,\nso this little calculation is necessary"
            # "all washing states are pricipally identical"
            n118 = call "Car Wash Timing (SubVI).vi"("Function"=enum16{"Reset Time", "Time Elapsed"}."Time Elapsed", "error in (no error)"=w448, "Time to Wait (s)"=w454) -> ("error out"=w444:errorcluster, "Remaining Time"=w456:dbl, "Time elapsed ?"=w457:bool)  [unwired: 6 in]
            n119 = To Double Precision Float(number=w454) -> (double precision float=w455:dbl)
            n120 = Subtract(x=w455, y=w456) -> (x-y=w446:dbl)
            n121 = in-place {
              # "setting car wash indicators"
              n122 = in-place-cluster #9(w462) -> ()  [unwired: 9 out]
              n123 = in-place-cluster #9("Under Body Wash"=FALSE, "Bug Remover"=FALSE, "Pre-Soak"=FALSE, "High Pressure Wash"=FALSE, "Low Pressure Wax"=FALSE, "Spot Free Rinse"=FALSE, "Tire Shine Foam"=FALSE, "Air Dry"=TRUE, "Vehicle Out of Position"=FALSE) -> (w461:T2)
            }
            n124 = Less?(x=w446, y=0.2) -> (x < y?=w445:bool)
            n125 = case shown="True" w445 {
              tunnel: w444 -> [w467 w471]
              tunnel: [w467 w470] -> w443
              tunnel: w439 -> [w464 w469]
              tunnel: w442 -> [w466 _]
              tunnel: [w465 FALSE] -> w441
              frame False {
                # "... then we check it"
                n126 = Not Equal?(x=w466, y=w464) -> (x != y?=w465:bool)
              }
              frame True {
                # "First, we set the car position ..."
                n127 = property on="Car Position Slider" class="Slide (strict)"(error in=w471, "Value"=w469) -> (error out=w470:errorcluster)  [unwired: 1 in, 1 out]
              }
            }
            n128 = Select(t=w458, s=w457, f=w440) -> (s? t:f=w450:T3)
            n129 = Select(t=w449, s=w441, f=w450) -> (s? t:f=w451:T3)
          }
          frame "Out of Position" {
            # "checking, if the vehicle is\nmoved back to the target\nstation, then return"
            # "all washing states are pricipally identical"
            n130 = in-place {
              # "setting car wash indicators"
              n131 = in-place-cluster #10(w493) -> ()  [unwired: 9 out]
              n132 = in-place-cluster #10("Under Body Wash"=FALSE, "Bug Remover"=FALSE, "Pre-Soak"=FALSE, "High Pressure Wash"=FALSE, "Low Pressure Wax"=FALSE, "Spot Free Rinse"=FALSE, "Tire Shine Foam"=FALSE, "Air Dry"=FALSE, "Vehicle Out of Position"=TRUE) -> (w492:T2)
            }
            n133 = Not Equal?(x=w483, y=w481) -> (x != y?=w482:bool)
            n134 = Select(t=Car_Wash_States."Out of Position" ("if time elapsed:"), s=w482, f=w484) -> (s? t:f=w486:T3)
          }
          frame "Wash Finished" {
            w507 = u8 4 items=["Entry", "Station 1", "Station 2", "Station 3", "Exit"] ("Car Position Slider")
            # "all washing states are pricipally identical"
            n135 = in-place {
              # "setting car wash indicators"
              n136 = in-place-cluster #11(w517) -> ()  [unwired: 9 out]
              n137 = in-place-cluster #11("Under Body Wash"=FALSE, "Bug Remover"=FALSE, "Pre-Soak"=FALSE, "High Pressure Wash"=FALSE, "Low Pressure Wax"=FALSE, "Spot Free Rinse"=FALSE, "Tire Shine Foam"=FALSE, "Air Dry"=FALSE, "Vehicle Out of Position"=TRUE) -> (w516:T2)
            }
            n138 = property on="Car Position Slider" class="Slide (strict)"(error in=w511) -> (error out=w505:errorcluster, "Value"=w508:u8)  [unwired: 1 in, 1 out]
            n139 = Equal?(x=w508, y=w507) -> (x = y?=w506:bool)
            n140 = Select(t=Car_Wash_States."Initialize" ("if time elapsed:"), s=w506, f=Car_Wash_States."Wash Finished" ("t")) -> (s? t:f=w512:T3)
          }
          frame "Stop" {
            w531 = T3[] [] items=["Initialize", "Customer Select", "Create Wash Process", "Reset Timer", "Under Body Wash", "Bug Remover", "Pre-Soak", "High Pressure Wash", "Low Pressure Wax", "Spot Free Rinse", "Tire Shine Foam", "Air Dry", "Out of Position", "Wash Finished", "Stop"]
            w538 = u8 0 items=["Entry", "Station 1", "Station 2", "Station 3", "Exit"] ("Car Position Slider")
            w539 = T2 {"Under Body Wash"=FALSE, "Bug Remover"=FALSE, "Pre-Soak"=FALSE, "High Pressure Wash"=FALSE, "Low Pressure Wax"=FALSE, "Spot Free Rinse"=FALSE, "Tire Shine Foam"=FALSE, "Air Dry"=FALSE, "Vehicle Out of Position"=FALSE}  # Car Wash Indicators
            # "we re-initialize all values of controls and indicators to their defaults"
            # "(L.9)"
            # "Stopping the program, resetting controls and indicators"
            n141 = control-ref of="This VI"() -> (w537:refnum<vi>)
            n142 = invoke class="VI" method="Default Vals.Reinit All"(reference=w537, error in=w534) -> (reference out=w536:refnum<vi>, error out=w535:errorcluster)  [unwired: 1 in, 1 out]
            n143 = Close Reference(reference=w536, error in (no error)=w535) -> (error out=w533:errorcluster)
            n144 = property on="Car Position Slider" class="Slide (strict)"(error in=w533, "Value"=w538) -> (error out=w530:errorcluster)  [unwired: 1 in, 1 out]
            n145 = property on="Wash Options" class="Clust (strict)"(error in=w530, "DisabledEnum"=T4."Enabled" ("Disabled")) -> (error out=w529:errorcluster)  [unwired: 1 in, 1 out]
          }
        }
        "Elapsed Time" <- w26
        "Car Wash Indicators" <- w34
        "Wash Entry" <- w32
        n146 = Equal?(x=w31, y=Car_Wash_States."Stop") -> (x = y?=w40:bool)
        n147 = Wait (ms)(milliseconds to wait=u32 50) -> ()  [unwired: 1 out]
      }
    }
    frame Error {
      # "do nothing"
    }
  }
  "error out" <- w1
  n148 = call <vilib>:"Simple Error Handler.vi"("error in (no error)"=w1) -> ()  [unwired: 4 in, 5 out]
